vi "test-function.vi"() -> ()   [LabVIEW 2017]
uses:
  CBB/ReadAllData.vi
  CBB/CreatTable.vi
  CBB/UpdateAllData.vi
  CBB/ClearTable.vi
  CBB/DropTable.vi
  CBB/RenameTable.vi
  CBB/DeleteRow.vi
  CBB/InsertRowData.vi
  CBB/UpdateOneData.vi
  CBB/UpdateDatas.vi
  SQLite.lvlib
panel:
  in  "InsertData":string[](array[string])
  in  "选项卡控件":enum32{"选项卡 1", "选项卡 2"}(tab)
  in  "Table Name":string
  in  "data-input":string[][](table)
  in  "退出":bool
  in  "执行":bool
  in  "项目选择":T1
  out "输出参数集合":T2
  in  "DbPath":path
  in  "Columns input":string[](array[string])
  in  "UpDateData":string
  in  "UpDateCol":string
  in  "Frist ColData":string
  in  "NewTableName":string
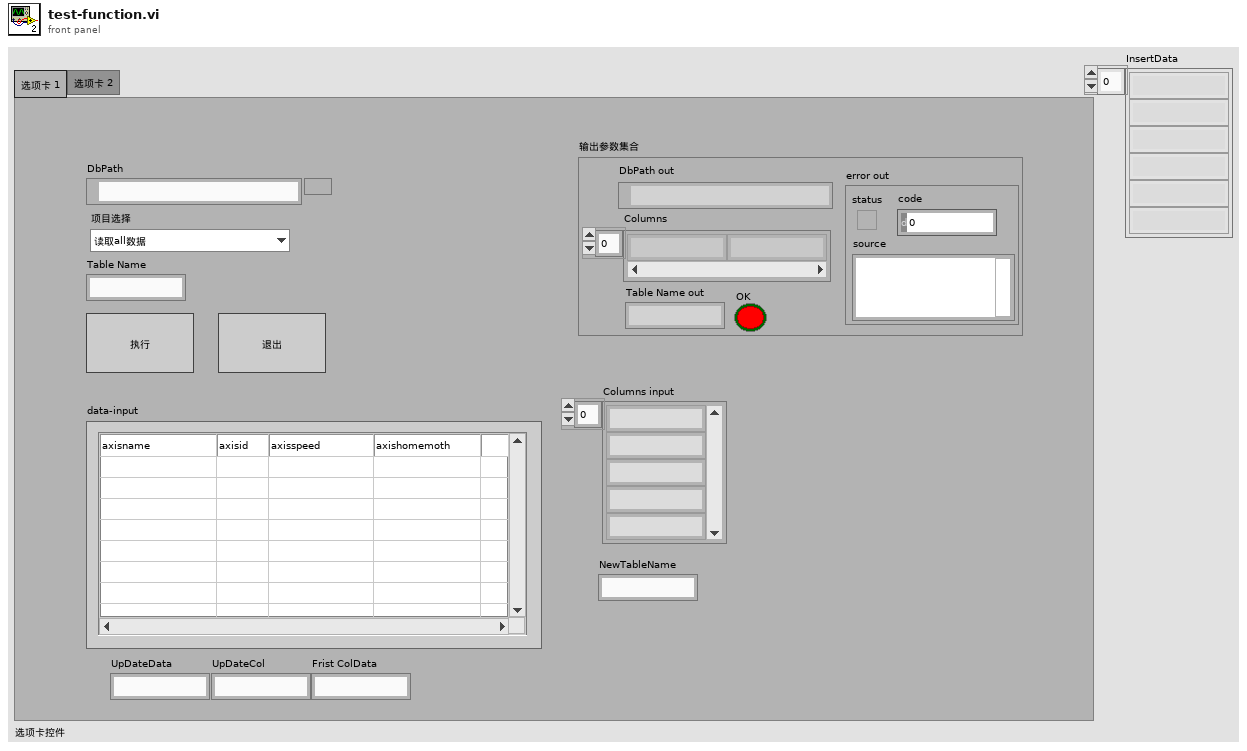
[diagram p1: front panel]
types:
  T1 = typedef "test项目选择.ctl" = enum16{"读取all数据", "创建新的table", "更新all表内容", "清除table内容", "删除table", "重命名table", "删除一行", "插入一行", "更新一个col", "更新一组col", "ListTable"}
  T2 = typedef "输出参数集合.ctl" = cluster{"DbPath out":path, "Columns":string[], "Table Name out":string, "OK":bool, "error out":errorcluster}
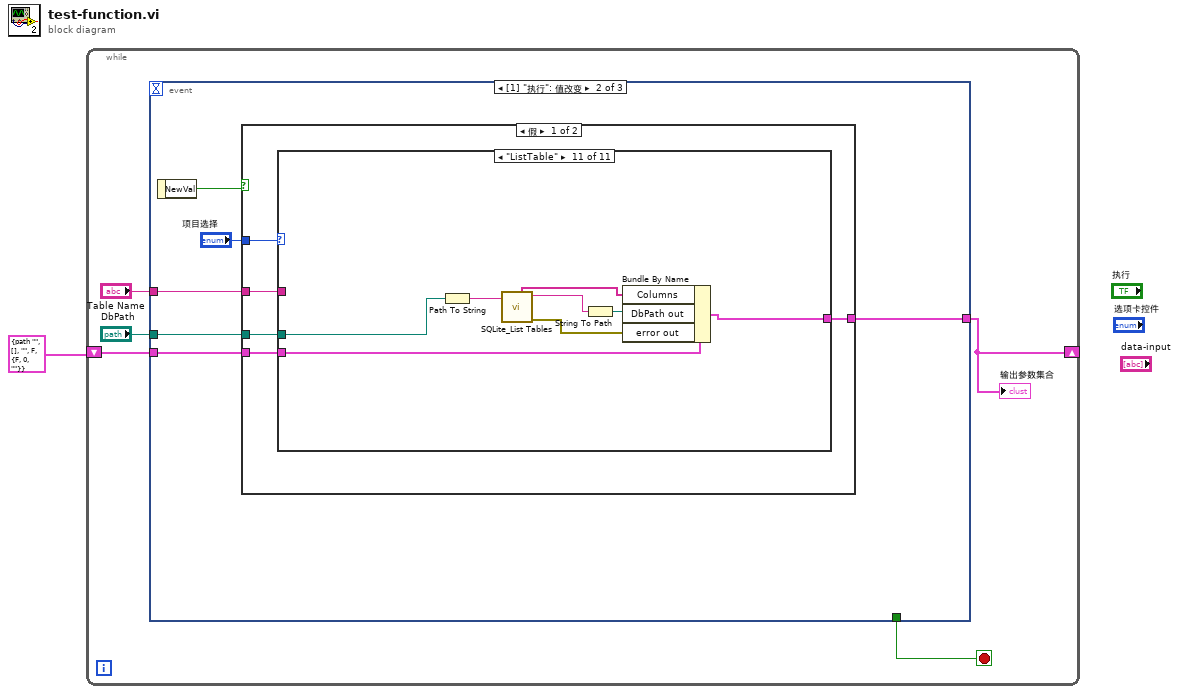
[diagram p0: block diagram]
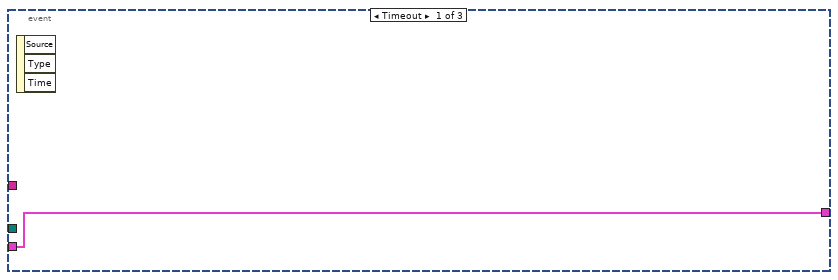
[diagram p2: hidden frame]
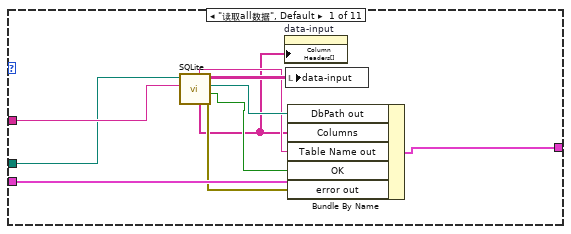
[diagram p3: hidden frame]
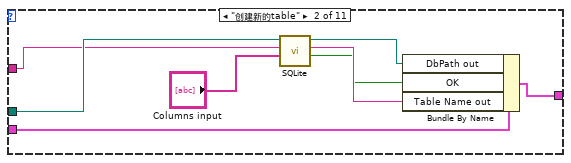
[diagram p4: hidden frame]
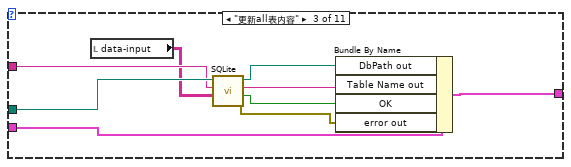
[diagram p5: hidden frame]
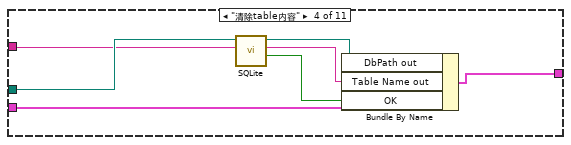
[diagram p6: hidden frame]
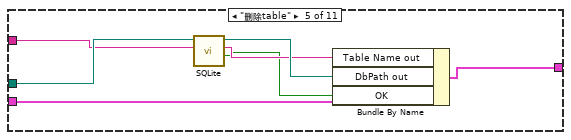
[diagram p7: hidden frame]
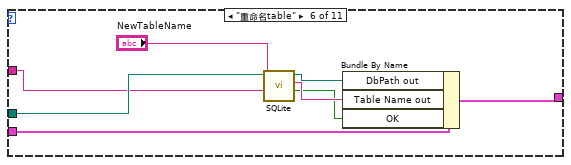
[diagram p8: hidden frame]
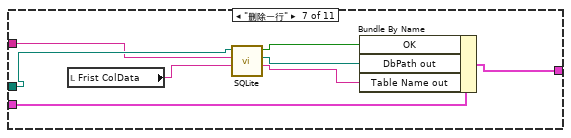
[diagram p9: hidden frame]
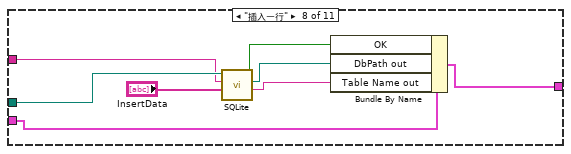
[diagram p10: hidden frame]
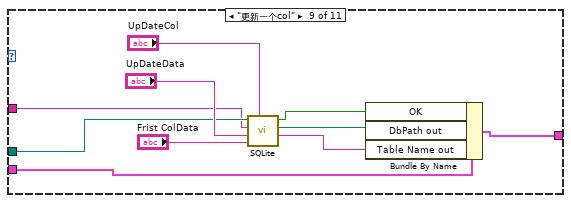
[diagram p11: hidden frame]
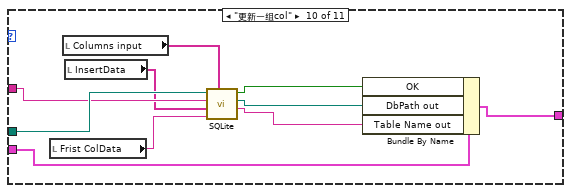
[diagram p12: hidden frame]
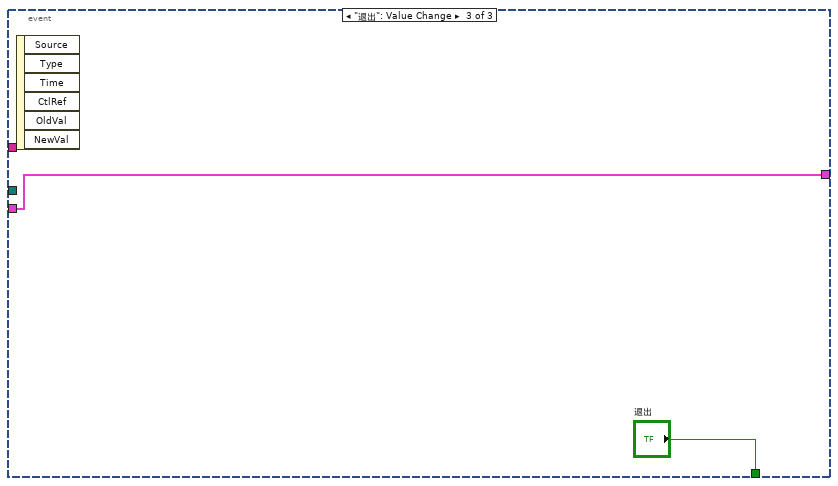
[diagram p14: hidden frame]
diagram:
  n1 = while {
    shift-right: [w3] -> _
    shift-left: T2 {"DbPath out"=path "", "Columns"=[], "Table Name out"="", "OK"=FALSE, "error out"={"status"=FALSE, "code"=0, "source"=""}} ("输出参数集合") -> [w5]
    stop <- w6 stop-if-true
    n2 = event shown="[1] \"执行\": 值改变" {
      selector: _ -> [_ _ _]
      dyn-events: _ -> [_ _ _]
      timeout: _ -> [_ _ _]
      tunnel: [_ _ "退出"] -> w6
      tunnel: w5 -> [w7 w11 w113]
      tunnel: "Table Name" -> [_ w10 _]
      tunnel: [w7 w9 w113] -> w3
      tunnel: "DbPath" -> [_ w8 _]
      event Timeout {
        n3 = event-data() -> ()  [unwired: 1 in, 3 out]
      }
      event "执行": Value Change {
        n4 = event-data() -> ("NewVal"=w13:bool)  [unwired: 1 in]
        n5 = case shown="假" w13 {
          tunnel: "项目选择" -> [w18 _]
          tunnel: w11 -> [w17 w112]
          tunnel: w10 -> [w16 _]
          tunnel: [w15 w112] -> w9
          tunnel: w8 -> [w14 _]
          frame False {
            n6 = case shown="\"ListTable\"" w18 {
              tunnel: w17 -> [w26 w33 w42 w50 w59 w64 w73 w78 w90 w98 w109]
              tunnel: w16 -> [w28 w35 w44 w51 w56 w66 w74 w76 w84 w102 _]
              tunnel: [w21 w29 w38 w46 w58 w60 w69 w77 w86 w94 w104] -> w15
              tunnel: w14 -> [w19 w36 w45 w52 w57 w67 w75 w79 w85 w103 w111]
              frame "读取all数据", Default {
                n7 = call-poly "SQLite.vi"("Table Name"=w28, "DbPath"=w19) -> ("error out"=w22:errorcluster, "OK"=w23:bool, "DbPath out"=w25:path, "Results"=w27:string[][], "Columns"=w20:string[], "Table Name out"=w24:string)  [unwired: 4 in]
                n8 = property on="data-input" class="Tbl (严格)"("Column Headers[]"=w20) -> ()  [unwired: 2 in, 2 out]
                n9 = local write "data-input"(w27) -> ()
                n10 = Bundle By Name(cluster=w26, "DbPath out"=w25, "Columns"=w20, "Table Name out"=w24, "OK"=w23, "error out"=w22) -> (w21:T2)
              }
              frame "创建新的table" {
                n11 = call-poly "SQLite.vi"("Columns"="Columns input", "Table Name"=w35, "DbPath"=w36) -> ("OK"=w30:bool, "Table Name out"=w31:string, "DbPath out"=w32:path)  [unwired: 6 in]
                n12 = Bundle By Name(cluster=w33, "DbPath out"=w32, "OK"=w30, "Table Name out"=w31) -> (w29:T2)
              }
              frame "更新all表内容" {
                n13 = local read "data-input"() -> (w43:string[][])
                n14 = call-poly "SQLite.vi"("AllData"=w43, "Table Name"=w44, "DbPath"=w45) -> ("error out"=w37:errorcluster, "OK"=w39:bool, "Table Name out"=w40:string, "DbPath out"=w41:path)  [unwired: 5 in]
                n15 = Bundle By Name(cluster=w42, "DbPath out"=w41, "Table Name out"=w40, "OK"=w39, "error out"=w37) -> (w38:T2)
              }
              frame "清除table内容" {
                n16 = call-poly "SQLite.vi"("Table Name"=w51, "Path"=w52) -> ("OK？"=w47:bool, "Table Name"=w48:string, "Path"=w49:path)  [unwired: 6 in, 1 out]
                n17 = Bundle By Name(cluster=w50, "DbPath out"=w49, "Table Name out"=w48, "OK"=w47) -> (w46:T2)
              }
              frame "删除table" {
                n18 = call-poly "SQLite.vi"("Table Name"=w56, "Path"=w57) -> ("OK？"=w53:bool, "Table Name"=w54:string, "Path"=w55:path)  [unwired: 7 in]
                n19 = Bundle By Name(cluster=w59, "Table Name out"=w54, "DbPath out"=w55, "OK"=w53) -> (w58:T2)
              }
              frame "重命名table" {
                n20 = call-poly "SQLite.vi"("OldTableName"=w66, "NewTableName"="NewTableName", "Path"=w67) -> ("OK？"=w61:bool, "Table Name"=w62:string, "Path"=w63:path)  [unwired: 6 in]
                n21 = Bundle By Name(cluster=w64, "DbPath out"=w63, "Table Name out"=w62, "OK"=w61) -> (w60:T2)
              }
              frame "删除一行" {
                n22 = local read "Frist ColData"() -> (w68:string)
                n23 = call-poly "SQLite.vi"("Frist ColData"=w68, "Table Name"=w74, "DbPath"=w75) -> ("Table Name out"=w70:string, "DbPath out"=w72:path, "OK"=w71:bool)  [unwired: 6 in]
                n24 = Bundle By Name(cluster=w73, "OK"=w71, "DbPath out"=w72, "Table Name out"=w70) -> (w69:T2)
              }
              frame "插入一行" {
                n25 = call-poly "SQLite.vi"("InsertData"="InsertData", "Table Name"=w76, "DbPath"=w79) -> ("Table Name out"=w80:string, "DbPath out"=w82:path, "OK"=w81:bool)  [unwired: 6 in]
                n26 = Bundle By Name(cluster=w78, "OK"=w81, "DbPath out"=w82, "Table Name out"=w80) -> (w77:T2)
              }
              frame "更新一个col" {
                n27 = call-poly "SQLite.vi"("UpDateCol"="UpDateCol", "Frist ColData"="Frist ColData", "UpDateData"="UpDateData", "Table Name"=w84, "DbPath"=w85) -> ("Table Name out"=w87:string, "DbPath out"=w89:path, "OK"=w88:bool)  [unwired: 4 in]
                n28 = Bundle By Name(cluster=w90, "OK"=w88, "DbPath out"=w89, "Table Name out"=w87) -> (w86:T2)
              }
              frame "更新一组col" {
                n29 = local read "Frist ColData"() -> (w100:string)
                n30 = local read "Columns input"() -> (w99:string[])
                n31 = local read "InsertData"() -> (w101:string[])
                n32 = call-poly "SQLite.vi"("UpDateCol"=w99, "Frist ColData"=w100, "UpDateData"=w101, "Table Name"=w102, "DbPath"=w103) -> ("Table Name out"=w95:string, "DbPath out"=w97:path, "OK"=w96:bool)  [unwired: 4 in]
                n33 = Bundle By Name(cluster=w98, "OK"=w96, "DbPath out"=w97, "Table Name out"=w95) -> (w94:T2)
              }
              frame "ListTable" {
                n34 = Path To String(path=w111) -> (string=w110:string)
                n35 = call "SQLite_List Tables.vi"("DB Path"=w110) -> ("Tables"=w106:string[], "DB Path Out"=w107:string, "error out"=w105:errorcluster)  [unwired: 7 in]
                n36 = String To Path(string=w107) -> (path=w108:path)
                n37 = Bundle By Name(cluster=w109, "Columns"=w106, "DbPath out"=w108, "error out"=w105) -> (w104:T2)
              }
            }
          }
          frame True {
          }
        }
      }
      event "退出": Value Change {
        n38 = event-data() -> ()  [unwired: 1 in, 6 out]
      }
    }
    "输出参数集合" <- w3
  }
